vi "ErrorManager_Loop.vi"(9 "Stop":bool, 10 "user event in":refnum<user-event>, 11 "queue error in":refnum<queue>) -> ()   [LabVIEW 2024, in "Error.lvlib"]
uses:
  Error.lvlib
  ErrorModel/ErrorMessage.ctl
  ErrorModel/ErrorSeverity.ctl
  ErrorModel/ErrorUIEvent.ctl
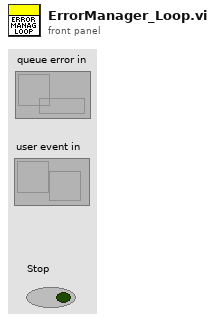
[diagram p1: front panel]
types:
  T1 = typedef "Error.lvlib/ErrorUIEvent.ctl" = cluster{"Time Stamp":timestamp, "ErrorSeverity":T2, "Source":string, "Message":string, "Code":i32}
  T2 = typedef "Error.lvlib/ErrorSeverity.ctl" = enum16{"INFO", "WARNING", "CRITICAL"}
  T3 = typedef "Error.lvlib/ErrorMessage.ctl" = cluster{"Time Stamp":timestamp, "Source":string, "Code":i32, "Message":string, "ErrorSeverity":T2}
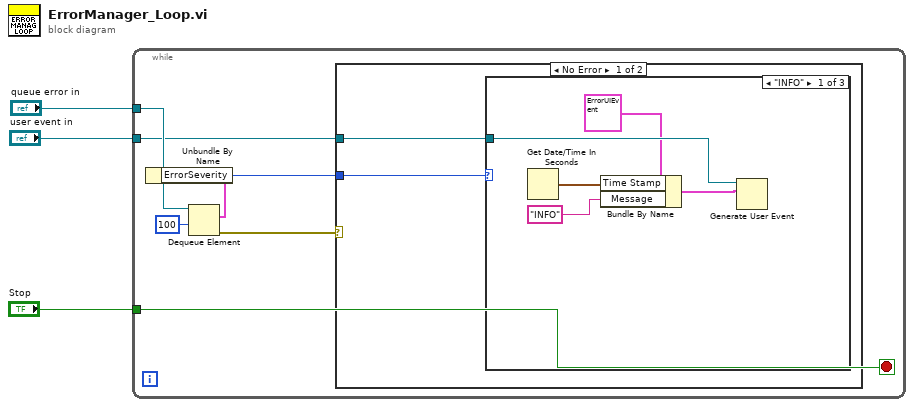
[diagram p0: block diagram]
diagram:
  n1 = while {
    tunnel: "queue error in" -> [w10]
    tunnel: "Stop" -> [w6]
    tunnel: "user event in" -> [w5]
    stop <- w6 stop-if-true
    n2 = Dequeue Element(queue=w10, timeout in ms (-1)=100) -> (element=w8:T3, error out=w4:errorcluster)  [unwired: 1 in, 2 out]
    n3 = Unbundle By Name(w8) -> ("ErrorSeverity"=w7:T2)
    n4 = case shown="No Error" w4 {
      tunnel: w7 -> [w12 _]
      tunnel: w5 -> [w11 _]
      frame No Error {
        n5 = case shown="\"INFO\"" w12 {
          tunnel: w11 -> [w17 _ _]
          frame "INFO" {
            n6 = Get Date/Time In Seconds() -> (seconds since 1Jan1904=w15:timestamp)
            n7 = Bundle By Name(cluster=T1 {"Time Stamp"=timestamp(0 s since 1904-01-01), "ErrorSeverity"=enum."INFO", "Source"="", "Message"="", "Code"=0} ("event data"), "Time Stamp"=w15, "Message"="INFO") -> (w14:T1)
            n8 = Generate User Event(user event=w17, event data cluster=w14) -> ()  [unwired: 2 in, 2 out]
          }
          frame "WARNING" {
          }
          frame "CRITICAL" {
          }
        }
      }
      frame Error {
      }
    }
  }
